vi "Set-control-enable-multiple.vi"(8 "error in (no error)":errorcluster, 9 "Enable?":bool, 10 "Control names":T1[](array[typedef]), 11 "UI ref. in":refnum<data-value>) -> (0 "error out":errorcluster, 3 "UI ref.":refnum<data-value>)   [LabVIEW 2013, in "CameraVision.lvlib" / "CV-UI.lvclass"]
uses:
  CV-UI.lvclass
  Control-names.ctl
  CV-UI.lvclass/CV-UI.ctl
  Read Control refs.vi
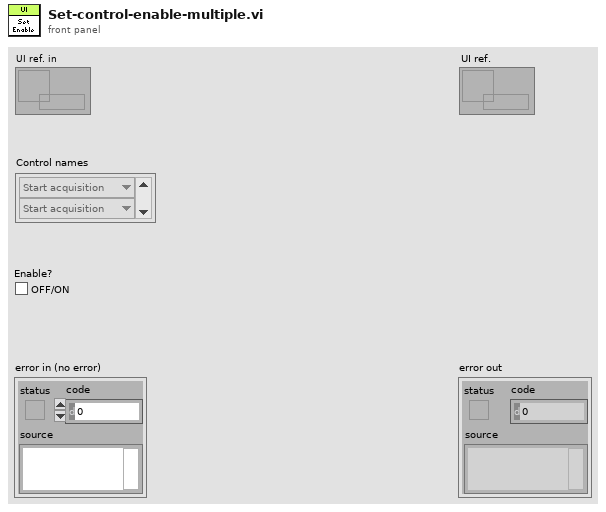
[diagram p1: front panel]
types:
  T1 = typedef "CameraVision.lvlib/CV-UI.lvclass/Control-names.ctl" = enum16{"Start acquisition", "Activate", "Stop acquisition", "Settings type", "Load settings", "Save settings", "Import images", "Camera selector", "Image type selector", "Batch browser", "Image refresh", "Parameter tabs", "Displays", "Processing tabs", "Processing selector", "Map characteristic", "Show info", "Manual trigger"}
  T2 = enum8{"Enabled", "Disabled", "Disabled and Grayed Out"}
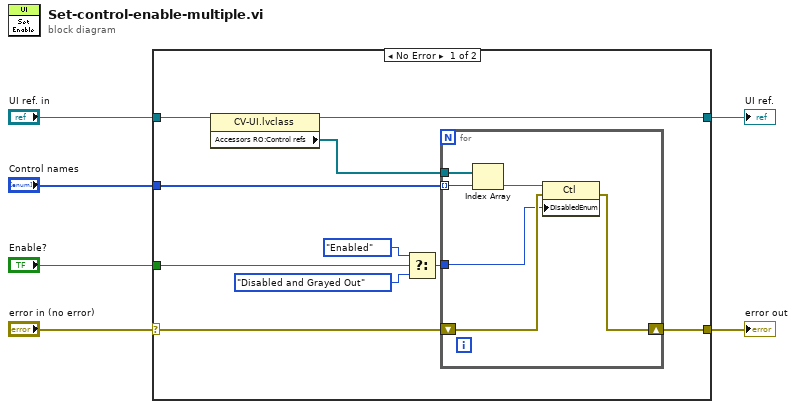
[diagram p0: block diagram]
diagram:
  n1 = case shown="No Error" "error in (no error)" {
    selector: "error in (no error)" -> [w11 w23]
    tunnel: [w13 w23] -> w5
    tunnel: [w12 w24] -> w3
    tunnel: "UI ref. in" -> [w16 w24]
    tunnel: "Control names" -> [w14 _]
    tunnel: "Enable?" -> [w10 _]
    frame No Error {
      n2 = property class="CV-UI.lvclass"(reference=w16) -> (reference out=w12:refnum<data-value>, "Accessors RO:Control refs"=w15:refnum<vi>[])  [unwired: 1 in, 1 out]
      n3 = Select(t=T2."Enabled" ("Disabled"), s=w10, f=T2."Disabled and Grayed Out" ("Disabled")) -> (s? t:f=w9:T2)
      n4 = for {
        tunnel: w15 -> [w22]
        tunnel: w14 -> [w21] mode=indexing
        tunnel: w9 -> [w17]
        shift-right: [w20] -> w13
        shift-left: w11 -> [w18]
        n5 = Index Array(array=w22, index=w21) -> (element=w19:refnum<vi>)
        n6 = property class="Ctl"(reference=w19, error in=w18, "DisabledEnum"=w17) -> (error out=w20:errorcluster)  [unwired: 1 out]
      }
    }
    frame Error {
    }
  }
  "error out" <- w5
  "UI ref." <- w3
